vi "New.vi"(8 "Error In":errorcluster, 11 "Key-Value Pairs":cluster{"Key":string, "Value":string}[](array[cluster])) -> (0 "Error Out":errorcluster, 3 "String":refnum<class "String.lvclass">)   [LabVIEW 2018, in "Toolkit.lvlib" / "Loaders.lvlib" / "String.lvclass"]
doc: "Creates a new String partial loader."
uses:
  String.lvclass
  String.lvclass/String.ctl
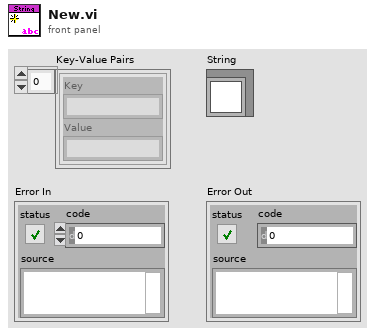
[diagram p1: front panel]
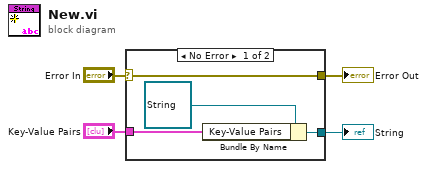
[diagram p0: block diagram]
diagram:
  n1 = case shown="No Error" "Error In" {
    selector: "Error In" -> [w5 w9]
    tunnel: "Key-Value Pairs" -> [w7 _]
    tunnel: [w6 _] -> w3
    tunnel: [w5 w9] -> w1
    frame No Error {
      n2 = Bundle By Name(cluster=refnum<class "String.lvclass"> refnum ("Toolkit.lvlib:Loaders.lvlib:String.lvclass"), "Key-Value Pairs"=w7) -> (w6:refnum<class "String.lvclass">)
    }
    frame Error {
    }
  }
  "String" <- w3
  "Error Out" <- w1
